vi "曲线处理C.vi"(7 "基值":sgl=2.55 format="%.2f", 8 "历史数据":sgl[](array[numeric]), 11 "力觉参数C":T1={"选择"=enum."Fx", "系数"=1.0, "上限"=4.3, "下限"=3.7, "Ymax"=50.0, "Ymin"=-50.0, "点数"=1000.0, "锁系数x"=1.0, "锁上限"=0.4, "锁下限"=0.6, "锁系数+"=1.0, "起点"=0.0, "终点"=0.0, "锁起点"=0.0, "锁终点"=0.0} {"锁终点" format="%.2f"; "锁起点" format="%.2f"; "终点" format="%.2f"; "起点" format="%.2f"; "锁系数+" format="%.3f"; "锁下限" format="%.2f"; "锁上限" format="%.2f"; "锁系数x" format="%.3f"; "下限" format="%.2f"; "上限" format="%.2f"; "系数" format="%.3f"}) -> (0 "范围内?":bool, 3 "曲线数组":sgl[](array[numeric]), 4 "值显示":string)   [LabVIEW 2018]
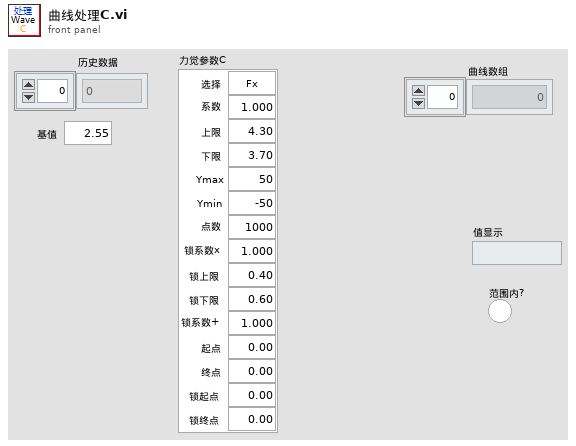
[diagram p1: front panel]
types:
  T1 = cluster{"选择":enum16{"Fx", "Fy", "Fz", "Mx", "My", "Mz"}, "系数":sgl, "上限":sgl, "下限":sgl, "Ymax":dbl, "Ymin":dbl, "点数":dbl, "锁系数x":sgl, "锁上限":sgl, "锁下限":sgl, "锁系数+":sgl, "起点":dbl, "终点":dbl, "锁起点":dbl, "锁终点":dbl}
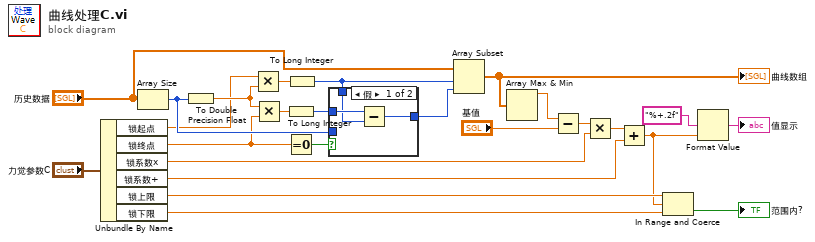
[diagram p0: block diagram]
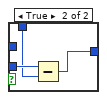
[diagram p2: hidden frame]
diagram:
  n1 = Unbundle By Name("力觉参数C") -> ("锁起点"=w1:dbl, "锁终点"=w2:dbl, "锁系数x"=w9:sgl, "锁系数+"=w7:sgl, "锁上限"=w6:sgl, "锁下限"=w5:sgl)
  n2 = Array Size(array="历史数据") -> (size(s)=w16:i32)
  n3 = To Double Precision Float(number=w16) -> (double precision float=w14:dbl)
  n4 = Multiply(x=w1, y=w14) -> (x*y=w18:dbl)
  n5 = Multiply(x=w14, y=w2) -> (x*y=w17:dbl)
  n6 = To Long Integer(number=w17) -> (32bit integer=w15:i32)
  n7 = Equal To 0?(x=w2) -> (x = 0?=w19:bool)
  n8 = To Long Integer(number=w18) -> (32bit integer=w12:i32)
  n9 = case shown="假" w19 {
    tunnel: w16 -> [_ w31]
    tunnel: w15 -> [w28 _]
    tunnel: w12 -> [w27 w30]
    tunnel: [w26 w29] -> w11
    frame False {
      n10 = Subtract(x=w28, y=w27) -> (x-y=w26:i32)
    }
    frame True {
      n11 = Subtract(x=w31, y=w30) -> (x-y=w29:i32)
    }
  }
  n12 = Array Subset(array="历史数据", index=w12, length=w11) -> (w24:sgl[])
  "曲线数组" <- w24
  n13 = Array Max & Min(array=w24) -> (max value=w23:sgl)  [unwired: 3 out]
  n14 = Subtract(x=w23, y="基值") -> (x-y=w10:sgl)
  n15 = Multiply(x=w10, y=w9) -> (x*y=w8:sgl)
  n16 = Add(x=w8, y=w7) -> (x+y=w4:sgl)
  n17 = In Range and Coerce(upper limit=w6, x=w4, lower limit=w5) -> (In Range?=→"范围内?":bool)  [unwired: 1 out]
  n18 = Format Value(format string="%+.2f" ("格式字符串"), value (0)=w4) -> (output string=→"值显示":string)  [unwired: 1 in]
